vi "read_params.vi"(8 "error in (no error)":errorcluster, 11 "GaussianProcessRegressor in":refnum<class "GaussianProcessRegressor.lvclass">) -> (0 "error out":errorcluster, 2 "params":T1={"alpha"={"alpha_type"="float", "alpha_float"=1e-10, "alpha_list"=[]}, "n_restarts_optimizer"=0.0, "normalize_y"=FALSE, "copy_X_train"=TRUE, "random_state"=0.0}, 3 "GaussianProcessRegressor out":refnum<class "GaussianProcessRegressor.lvclass">)   [LabVIEW 2020, in "GaussianProcessRegressor.lvclass"]
uses:
  GaussianProcessRegressor.lvclass
  Controls/gaussian_process_regressor_params.ctl
  GaussianProcessRegressor.lvclass/GaussianProcessRegressor.ctl
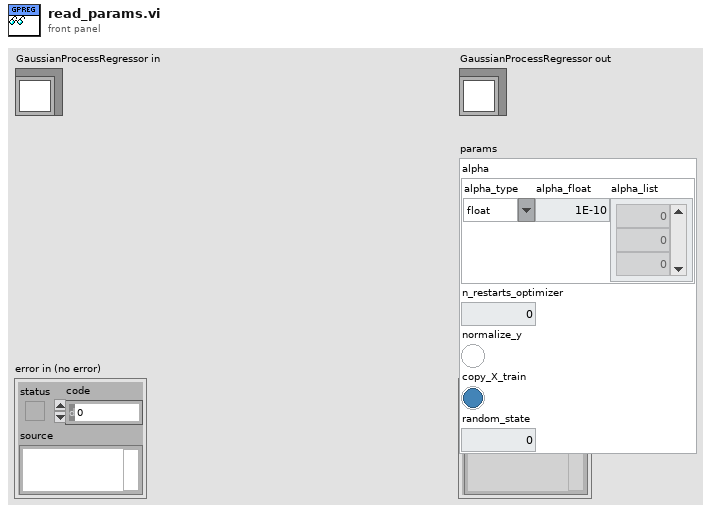
[diagram p1: front panel]
types:
  T1 = typedef "gaussian_process_regressor_params.ctl" = cluster{"alpha":cluster{"alpha_type":string, "alpha_float":dbl, "alpha_list":dbl[]}, "n_restarts_optimizer":dbl, "normalize_y":bool, "copy_X_train":bool, "random_state":dbl}
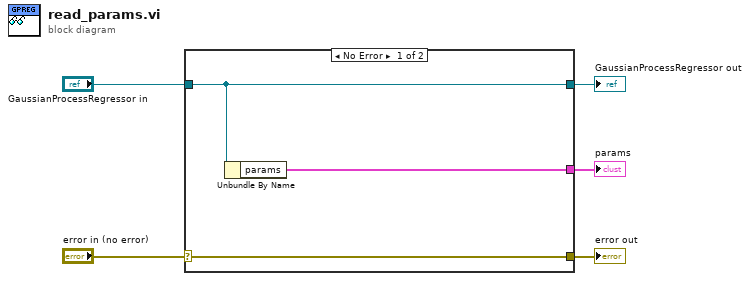
[diagram p0: block diagram]
diagram:
  n1 = case shown="No Error" "error in (no error)" {
    selector: "error in (no error)" -> [w8 w9]
    tunnel: [w8 w9] -> w4
    tunnel: [w7 w10] -> w2
    tunnel: "GaussianProcessRegressor in" -> [w7 w10]
    tunnel: [w6 _] -> w1
    frame No Error {
      n2 = Unbundle By Name(w7) -> ("params"=w6:T1)
    }
    frame Error {
    }
  }
  "error out" <- w4
  "GaussianProcessRegressor out" <- w2
  "params" <- w1
